vi "Calculate Line Reciprocal And Start.vi"(6 "y":sgl, 9 "x 2":sgl, 10 "y 2":sgl, 11 "x":sgl) -> (3 "Numeric":sgl)   [LabVIEW 2022 SP3]
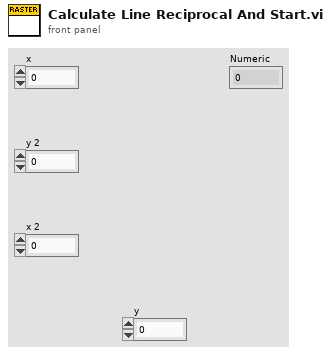
[diagram p1: front panel]
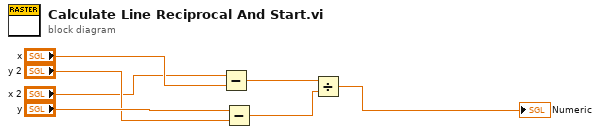
[diagram p0: block diagram]
diagram:
  n1 = Subtract(x="x 2", y="x") -> (x-y=w1:sgl)
  n2 = Subtract(x="y", y="y 2") -> (x-y=w2:sgl)
  n3 = Divide(x=w1, y=w2) -> (x/y=→"Numeric":sgl)
